vi "SPC_fill_memory.vi"(6 "Fill Value":u16 step=1, 7 "Block to be Filled":i32=-1 min=-1 max=65536 step=1, 8 "Error In":errorcluster, 9 "Page":i32=-1 min=-1 max=65536 step=1, 10 "Module No":i16 min=-1 max=7 step=1, 11 "DLL Path":path) -> (0 "Error Out":errorcluster, 1 "FunctionReturn":i16, 2 "Module No":i16, 3 "DLL Path":path)   [LabVIEW 2023]
doc: "The procedure is used to clear the measurement memory before a new measurement is started.\nIf 'mod_no' = -1 memory on all used SPC modules will be cleared, otherwise only on the module 'mod_no'.\nThe procedure fills a specified part of the SPC memory with the value 'fill_value'. \nTo provide correct memory access it is required that the function SPC_configure_memory be used ( normal operation modes) before the first call of SPC_fill_memory and always after setting ADC resolution parameter value. \nThe parameter 'block' can range from 0 to blocks_per_page - 1. \nIf the value '-1' is used all blocks on the specified page(s) are filled. \nThe parameter 'page' can vary from 0 to maxpage -1. \nIf the value '-1' is used all pages in current memory bank are filled.\n<b>Attention: </b>The procedure returns on success the number of the modules on which filling the memory was started but is still not finished. If this value is > 0, the function SPC_test_state must be called next to check whether the started filling process is already finished ( if the bit \nSPC_HFILL_NRDY is set in state, filling is not finished, see spcm_def.h for bit definition).\n\n<b>Note:</b> This VI is set to execute as preallocated clone to improve performance when run in parallel loops for multi module setups.\n\ninfo@becker-hickl.com"
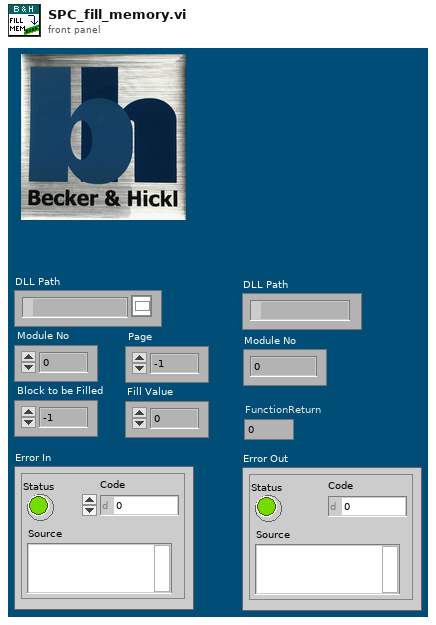
[diagram p1: front panel]
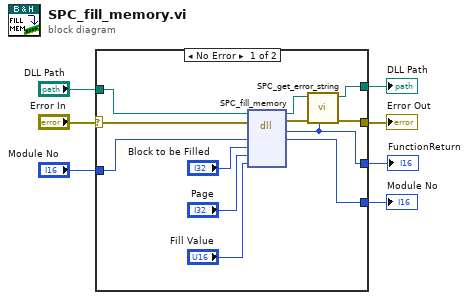
[diagram p0: block diagram]
diagram:
  n1 = case shown="No Error" "Error In" {
    selector: "Error In" -> [w15 w22]
    tunnel: "DLL Path" -> [w16 w21]
    tunnel: [w10 w21] -> w6
    tunnel: [w9 w22] -> w5
    tunnel: "Module No" -> [w14 w20]
    tunnel: [w13 w20] -> w2
    tunnel: [w8 _] -> w1
    frame No Error {
      n2 = dll-call lib="D:/spcm/lib/lab_view/lv10.0/spcm32.dll" fn="SPC_fill_memory"(path in=w16, error in=w15, "mod_no"=w14, "block"="Block to be Filled", "page"="Page", "fill_value"="Fill Value") -> (path out=w11:path, error out=w12:errorcluster, "return type"=w8:i16, "mod_no"=w13:i16)  [unwired: 4 in]
      n3 = call "SPC_get_error_string.vi"("ErrorID"=w8, "Error In"=w12, "DLL Path"=w11) -> ("Error Out"=w9:errorcluster, "DLL Path"=w10:path)  [unwired: 6 in, 1 out]
    }
    frame Error {
    }
  }
  "DLL Path" <- w6
  "Error Out" <- w5
  "Module No" <- w2
  "FunctionReturn" <- w1
